vi "Read TCPServer.vi"(8 "error in (no error)":errorcluster, 11 "MonoCommunicator in":refnum<class "MonoCommunicator.lvclass">) -> (0 "error out":errorcluster, 2 "TCPServer.lvclass":refnum<class "TCPServer.lvclass">, 3 "MonoCommunicator out":refnum<class "MonoCommunicator.lvclass">)   [LabVIEW 2016, in "MonoCommunicator.lvclass"]
uses:
  MonoCommunicator.lvclass
  ts_labview_tcp/TCPServer/TCPServer.lvclass
  MonoCommunicator.lvclass/MonoCommunicator.ctl
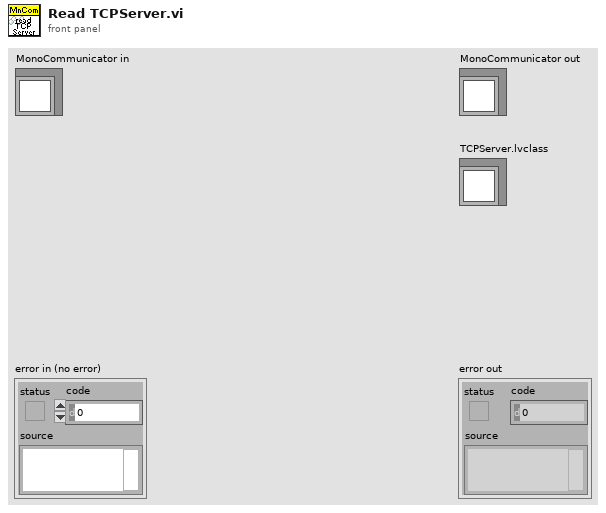
[diagram p1: front panel]
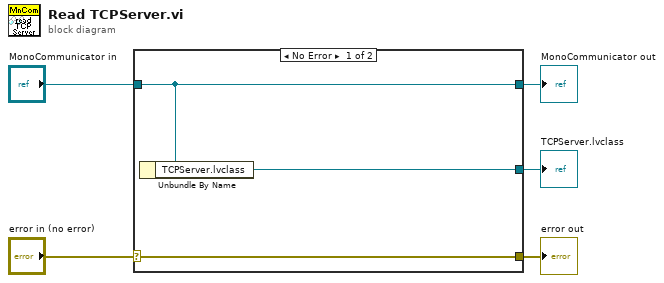
[diagram p0: block diagram]
diagram:
  n1 = case shown="No Error" "error in (no error)" {
    selector: "error in (no error)" -> [w8 w9]
    tunnel: [w8 w9] -> w4
    tunnel: [w7 w10] -> w2
    tunnel: "MonoCommunicator in" -> [w7 w10]
    tunnel: [w6 _] -> w1
    frame No Error {
      n2 = Unbundle By Name(w7) -> ("TCPServer.lvclass"=w6:refnum<class "TCPServer.lvclass">)
    }
    frame Error {
    }
  }
  "error out" <- w4
  "MonoCommunicator out" <- w2
  "TCPServer.lvclass" <- w1
